vi "CtrlHandlerDiagram.vi"(2 "Type":T1=enum."Value Change", 3 "Ctrl":refnum<vi>, 4 "Structure":refnum<vi>) -> (0 "Index":i32, 1 "Diagram":refnum<vi>)   [LabVIEW 2014]
uses:
  <vilib>/event_ctls.llb/lveventtype.ctl
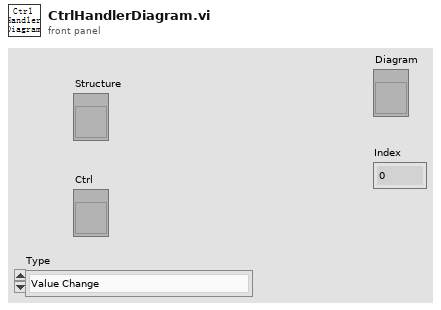
[diagram p1: front panel]
types:
  T1 = typedef "lveventtype.ctl" = enum32{"Null", "Timeout", "Annotation Menu Selection", "Annotation Menu Selection?", "App Instance Close", "App Instance Close?", "Autoscale Range Change", "Bookmark Info Change", "Cell Edit", "Cell Edit?", "Cursor Grab", "Cursor Grab?", "Cursor Menu Selection", "Cursor Menu Selection?", "Cursor Move", "Cursor Release", "Data Change", "Direction Change", "Display State Change", "Drag Ended", "Drag Enter", "Drag Leave", "Drag Over", "Drag Source Update", "Drag Starting", "Drag Starting?", "Drop", "Exec State Change", "Key Down", "Key Down?", "Key Repeat", "Key Repeat?", "Key Up", "Listbox Double Click", "Menu Activation?", "Menu Selection (App)", "Menu Selection? (App)", "Menu Selection (User)", "Mouse Down", "Mouse Down?", "Mouse Enter", "Mouse Leave", "Mouse Move", "Mouse Up", "Mouse Wheel", "NI Security User Change (App)", "Pane Size", "Panel Close", "Panel Close?", "Panel Resize", "Plot Attribute Change", "Scale Range Change", "Shortcut Menu Activation?", "Shortcut Menu Selection (App)", "Shortcut Menu Selection? (App)", "Shortcut Menu Selection (User)", "Tree Double Click", "Tree Drag", "Tree Drag?", "Tree Drop", "Tree Drop?", "Tree Item Close", "Tree Item Close?", "Tree Item Open", "Tree Item Open?", "User Event", "Value Change"}
  T2 = cluster{"Event Type":T1, "Reference":refnum<vi>, "Limit (-1=none)":i32, "Lock Panel?":bool}
  T3 = cluster{"Event Type":T1, "Reference":refnum<vi>, "Limit (-1=none)":i32, "Lock Panel?":bool}[]
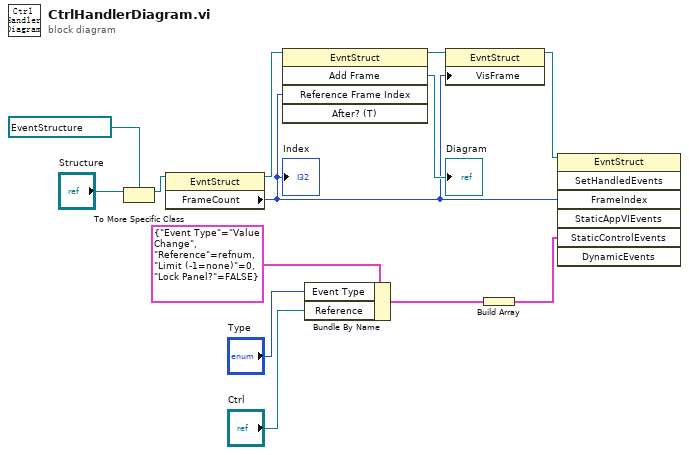
[diagram p0: block diagram]
diagram:
  n1 = To More Specific Class(target class=refnum<vi> refnum ("Structure"), reference="Structure") -> (specific class reference=w2:refnum<vi>)  [unwired: 1 in, 1 out]
  n2 = property class="EvntStruct"(reference=w2) -> (reference out=w13:refnum<vi>, "FrameCount"=w1:i32)  [unwired: 1 in, 1 out]
  "Index" <- w1
  n3 = invoke class="EvntStruct" method="Add Frame"(reference=w13, "Reference Frame Index"=w1) -> (reference out=w8:refnum<vi>, "Add Frame"=→"Diagram":refnum<vi>)  [unwired: 3 in, 3 out]
  n4 = Bundle By Name(cluster=T2 {"Event Type"=enum."Value Change", "Reference"=refnum, "Limit (-1=none)"=0, "Lock Panel?"=FALSE} ("Static Control Events"), "Event Type"="Type", "Reference"="Ctrl") -> (w9:T2)
  n5 = property class="EvntStruct"(reference=w8, "VisFrame"=w1) -> (reference out=w7:refnum<vi>)  [unwired: 1 in, 1 out]
  n6 = Build Array(w9) -> (w6:T3)
  n7 = invoke class="EvntStruct" method="SetHandledEvents"(reference=w7, "FrameIndex"=w1, "StaticControlEvents"=w6) -> ()  [unwired: 4 in, 7 out]
